vi "PDE_Tridiag Mtrx x Vec.vi"(8 "X":dbl[](array[numeric]), 9 "Super Diag":dbl[](array[numeric]), 10 "Diag":dbl[](array[numeric]), 11 "Sub Diag":dbl[](array[numeric])) -> (3 "Mtrx x X":dbl[](array[numeric]))   [LabVIEW 2020, in "NI_PDE.lvlib"]
uses:
  <vilib>/gmath/NI_PDE.lvlib
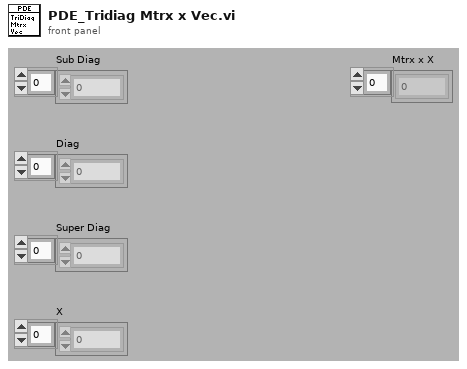
[diagram p1: front panel]
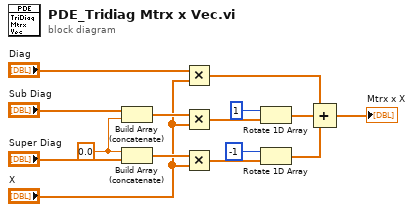
[diagram p0: block diagram]
diagram:
  w14 = 0.0
  n1 = Build Array (concatenate)("Sub Diag", w14) -> (w13:dbl[])
  n2 = Build Array (concatenate)(w14, "Super Diag") -> (w12:dbl[])
  n3 = Multiply(x="Diag", y="X") -> (x*y=w7:dbl[])
  n4 = Multiply(x=w13, y="X") -> (x*y=w6:dbl[])
  n5 = Multiply(x=w12, y="X") -> (x*y=w2:dbl[])
  n6 = Rotate 1D Array(1:w6, 2:1 ("n")) -> (0:w5:dbl[])
  n7 = Rotate 1D Array(1:w2, 2:-1 ("n")) -> (0:w1:dbl[])
  n8 = Compound Arithmetic op=ADD(w7, w5, w1) -> (→"Mtrx x X":dbl[])
